vi "Write VISA resource name.vi"(10 "VISA resource name":refnum<visa-resource-name>, 11 "Instrument in":refnum<class "Instrument.lvclass">) -> (3 "Instrument out":refnum<class "Instrument.lvclass">)   [LabVIEW 2020, in "Instrument.lvclass"]
uses:
  Instrument.lvclass
  Instrument.lvclass/Instrument.ctl
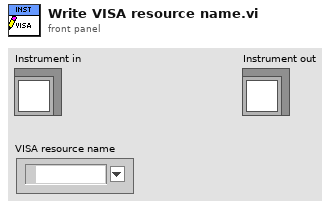
[diagram p1: front panel]
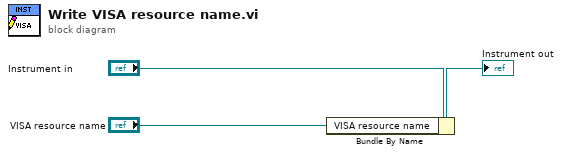
[diagram p0: block diagram]
diagram:
  n1 = Bundle By Name(cluster="Instrument in", "VISA resource name"="VISA resource name") -> (→"Instrument out":refnum<class "Instrument.lvclass">)
